vi "While Loop SCTL Benchmarking.vi"() -> ()   [LabVIEW 2010]
uses:
  <vilib>/Platform/TimedLoop/XDataNode/XDataNode.xnode
  <vilib>/Platform/TimedLoop/XDataNode/timing_clust.ctl
  <vilib>/Platform/TimedLoop/XDataNode/nitl_modes.ctl
  <vilib>/Platform/TimedLoop/XDataNode/wakeup.ctl
  <vilib>/Platform/TimedLoop/XDataNode/XDNodeRunTimeDep.lvlib
panel:
  out "Ticks (SCTL)":u32
  out "Avg Ticks (SCTL)":u32
  in  "Value A":i16
  in  "Value B":i16
  in  "Value C":i16
  in  "Value D":i16
  out "Average Value (ABCD)":i16
  out "Avg Ticks (While Loop)":u32
  out "Average Value (1234)":i16
  in  "Value 4":i16
  in  "Value 3":i16
  in  "Value 2":i16
  in  "Value 1":i16
  out "Ticks (While Loop)":u32
  # "While Loop Benchmark"
  # "SCTL Benchmark"
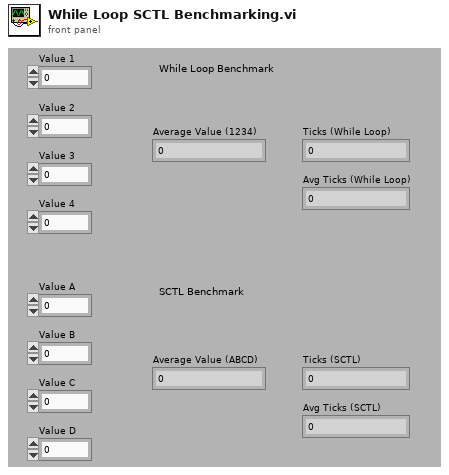
[diagram p1: front panel]
types:
  T1 = typedef "XDNodeRunTimeDep.lvlib/timing_clust.ctl" = cluster{"Expected End [f-1]":u64, "Actual End [f-1]":u64, "Finished Late? [f-1]":bool, "Expected End [i-1]":u64, "Actual End [i-1]":u64, "Finished Late? [i-1]":bool, "Expected Start [i]":u64, "Actual Start [i]":u64, "Expected Start [f]":u64, "Actual Start [f]":u64, "Source Name":string, "Structure Name":string, "Period":i64, "Deadline":i64, "Offset":i64, "Start":i64, "Priority":i32, "Timeout":i32, "Mode":T2, "Wakeup Reason":T3, "Error":errorcluster, "Source Type":string, "Secondary Source Type":string, "Global End Time":u64, "Global Start Time":u64, "Frame Duration":u64, "Iteration Duration":u64, "Assigned CPU":i32, "I/O Scan Engine Mode":u32}
  T2 = typedef "XDNodeRunTimeDep.lvlib/nitl_modes.ctl" = enum32{"No Change", "Process missed periods, maintain original phase", "Discard missed periods, maintain original phase", "Process missed periods, ignore original phase", "Discard missed periods, ignore original phase"}
  T3 = typedef "XDNodeRunTimeDep.lvlib/wakeup.ctl" = enum32{"Normal", "Aborted", "Asynchronous wakeup", "Timing source error", "Timed loop error", "Timeout"}
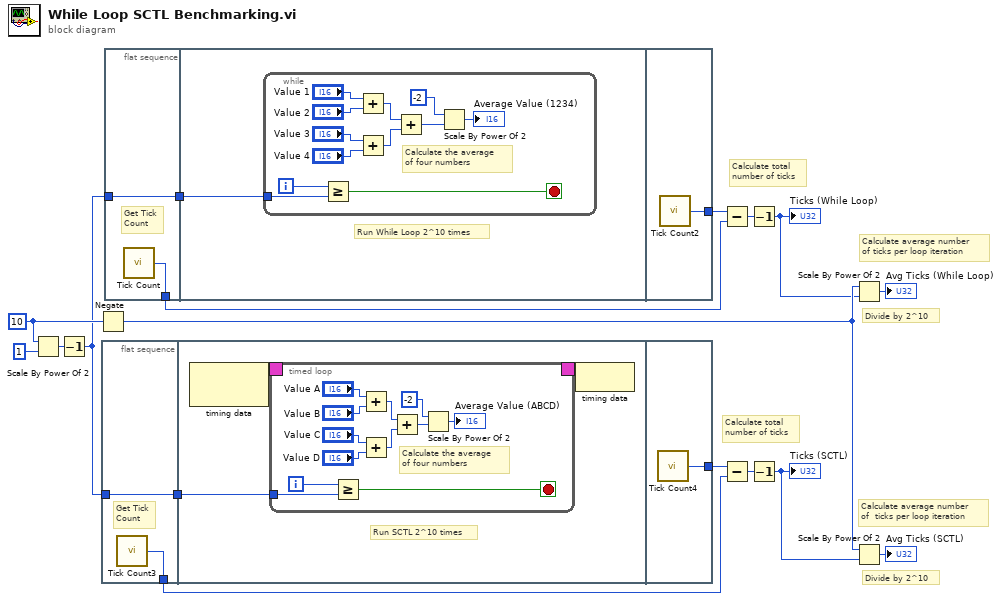
[diagram p0: block diagram]
diagram:
  w15 = 10 ("n")
  # "Calculate total\nnumber of ticks"
  # "Calculate total\nnumber of ticks"
  # "Calculate average number\nof  ticks per loop iteration"
  # "Divide by 2^10"
  # "Divide by 2^10"
  # "Calculate average number\nof ticks per loop iteration"
  n1 = Scale By Power Of 2(n=w15, x=1) -> (x*2^n=w16:i32)
  n2 = Decrement(x=w16) -> (x-1=w13:i32)
  n3 = Negate(x=w15) -> (-x=w7:i32)
  n4 = flat-sequence {
    tunnel: [w19] -> w14
    tunnel: w13 -> [w19]
    tunnel: [w18] -> w5
    tunnel: w14 -> [w20]
    tunnel: [w39] -> w6
    frame #0 {
      # "Get Tick\nCount"
      n5 = call "Tick Count3"() -> ("Tick Count(Ticks)"=w18:u32)
    }
    frame #1 {
      # "Run SCTL 2^10 times"
      n6 = node-c288() -> (w22:T1)  [unwired: 1 out]
      n7 = timed-loop {
        timing: w22 -> [_]
        timing-out: [_] -> w21
        tunnel: w20 -> [w23]
        i -> [w34]
        stop <- w33 stop-if-true
        # "Calculate the average\nof four numbers"
        n8 = Greater Or Equal?(x=w34, y=w23) -> (x >= y?=w33:bool)
        n9 = Add(x="Value A", y="Value B") -> (x+y=w28:i16)
        n10 = Add(x="Value C", y="Value D") -> (x+y=w27:i16)
        n11 = Add(x=w28, y=w27) -> (x+y=w25:i16)
        n12 = Scale By Power Of 2(n=-2, x=w25) -> (x*2^n=→"Average Value (ABCD)":i16)
      }
      n13 = node-c288(w21) -> ()
    }
    frame #2 {
      n14 = call "Tick Count4"() -> ("Tick Count(Ticks)"=w39:u32)
    }
  }
  n15 = flat-sequence {
    tunnel: w13 -> [w41]
    tunnel: [w41] -> w12
    tunnel: [w40] -> w10
    tunnel: w12 -> [w42]
    tunnel: [w55] -> w9
    frame #0 {
      # "Get Tick\nCount"
      n16 = call "Tick Count"() -> ("Tick Count(Ticks)"=w40:u32)
    }
    frame #1 {
      # "Run While Loop 2^10 times"
      n17 = while {
        tunnel: w42 -> [w43]
        i -> [w54]
        stop <- w53 stop-if-true
        # "Calculate the average\nof four numbers"
        n18 = Greater Or Equal?(x=w54, y=w43) -> (x >= y?=w53:bool)
        n19 = Add(x="Value 1", y="Value 2") -> (x+y=w48:i16)
        n20 = Add(x="Value 3", y="Value 4") -> (x+y=w47:i16)
        n21 = Add(x=w48, y=w47) -> (x+y=w45:i16)
        n22 = Scale By Power Of 2(n=-2, x=w45) -> (x*2^n=→"Average Value (1234)":i16)
      }
    }
    frame #2 {
      n23 = call "Tick Count2"() -> ("Tick Count(Ticks)"=w55:u32)
    }
  }
  n24 = Subtract(x=w9, y=w10) -> (x-y=w4:u32)
  n25 = Subtract(x=w6, y=w5) -> (x-y=w2:u32)
  n26 = Decrement(x=w4) -> (x-1=w3:u32)
  "Ticks (While Loop)" <- w3
  n27 = Decrement(x=w2) -> (x-1=w1:u32)
  "Ticks (SCTL)" <- w1
  n28 = Scale By Power Of 2(n=w7, x=w3) -> (x*2^n=→"Avg Ticks (While Loop)":u32)
  n29 = Scale By Power Of 2(n=w7, x=w1) -> (x*2^n=→"Avg Ticks (SCTL)":u32)
